vi "Child_s Second Move.vi"(10 "Old Light Sensor Array":i16[](array[numeric]), 11 "Current Image Array":i32[](array[numeric])) -> (2 "Image Value From Second Turn":i32, 3 "Output Image Array":i32[](array[numeric]))   [LabVIEW 2018]
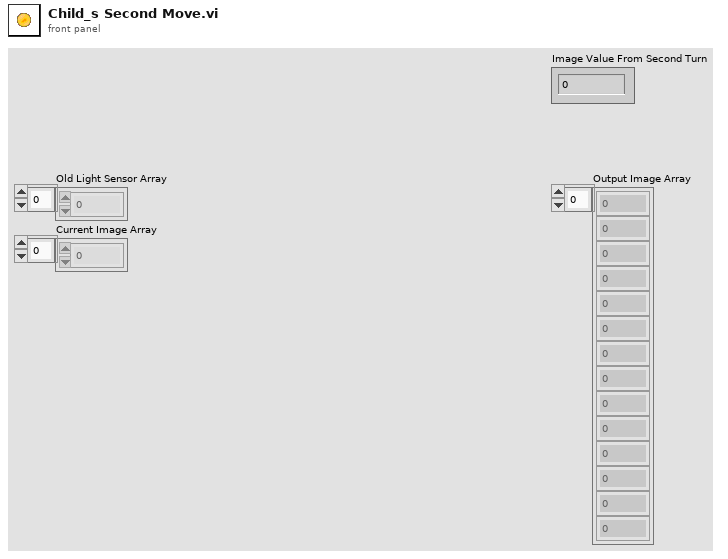
[diagram p1: front panel]
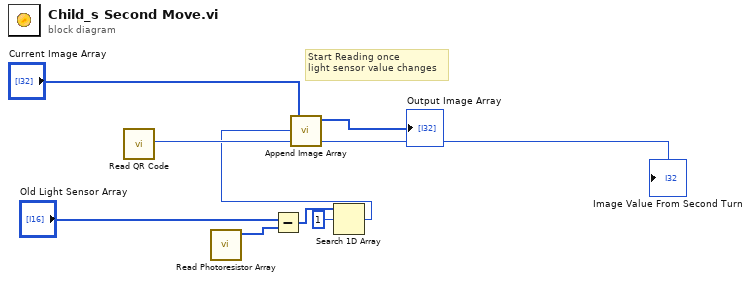
[diagram p0: block diagram]
diagram:
  # "Start Reading once \nlight sensor value changes"
  n1 = call "Read QR Code.vi"() -> ("Image Value"=w8:i32)  [unwired: 10 in, 1 out]
  "Image Value From Second Turn" <- w8
  n2 = call "Read Photoresistor Array.vi"() -> ("0, 1"=w7:i16[])  [unwired: 11 in]
  n3 = Subtract(x="Old Light Sensor Array", y=w7) -> (x-y=w6:i16[])
  n4 = Search 1D Array(1D array=w6, element=1) -> (index of element=w4:i32)  [unwired: 1 in]
  n5 = call "Append Image Array.vi"("index"=w4, "New Image Value"=w8, "Current Image Array"="Current Image Array") -> ("Output Image Array"=→"Output Image Array":i32[])  [unwired: 3 in]
